vi "Main Program.vi"() -> ()   [LabVIEW 2011]
panel:
  out "Mean Plot":dynamicdata(graph)
  out "Current data plot":cluster{"Y":dbl[], "Y":dbl[]}[](graph)
  in  "UP CONVERSION":enum32{"Set Position ", "Data Accusition"}(tab)
  in  "Position (units)":dbl
  in  "Velocity value (units/s) in":dbl
  out "Current position (units)":dbl
  out "Velocity value (units/s) out":dbl
  in  "stop":bool
  out "Position Time Zero":dbl
  in  "Velocity for detecting position zero":dbl
  in  "Set count 1":i32
  in  "Velocity 1":dbl
  in  "Step Size 1":dbl
  in  "Set count 2":i32
  in  "Velocity 2":dbl
  in  "Step Size 2":dbl
  in  "Set count 3":i32
  in  "Velocity 3":dbl
  in  "Step Size 3":dbl
  in  "Set count 4":i32
  in  "Velocity 4":dbl
  in  "Step Size 4":dbl
  in  "File Path":string="C:\\Users\\nshukla\\Desktop\\2\\"
  in  "Stop Taking Data":bool
  in  "Average file path":path
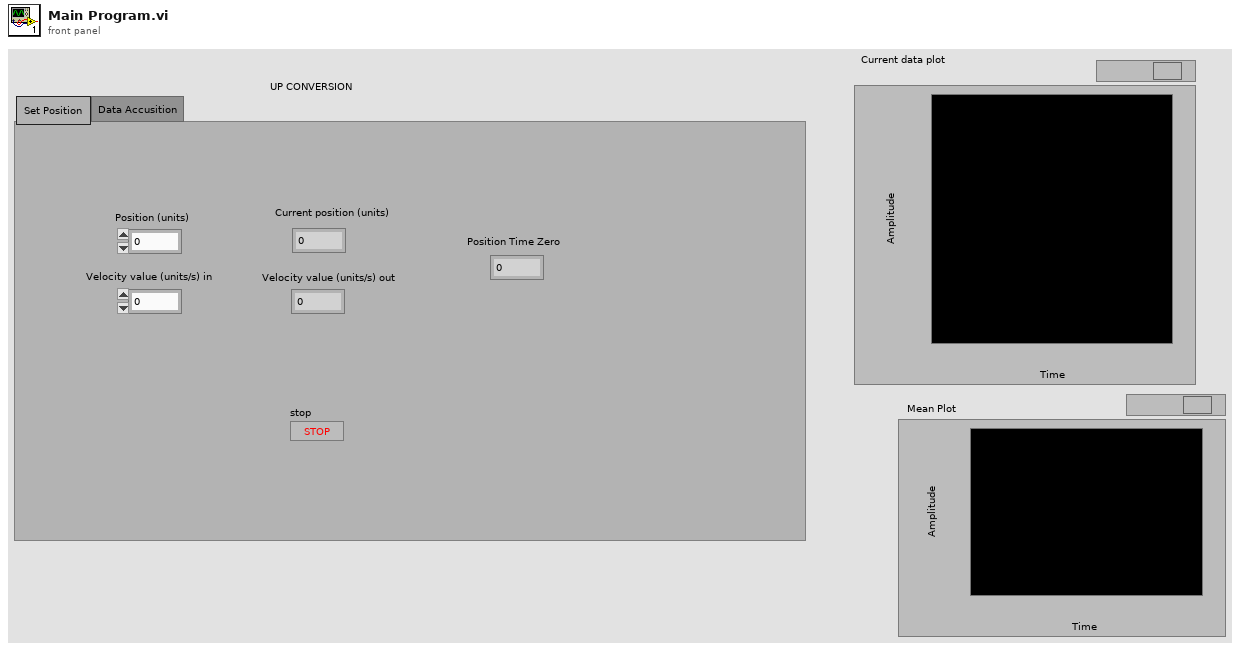
[diagram p1: front panel]
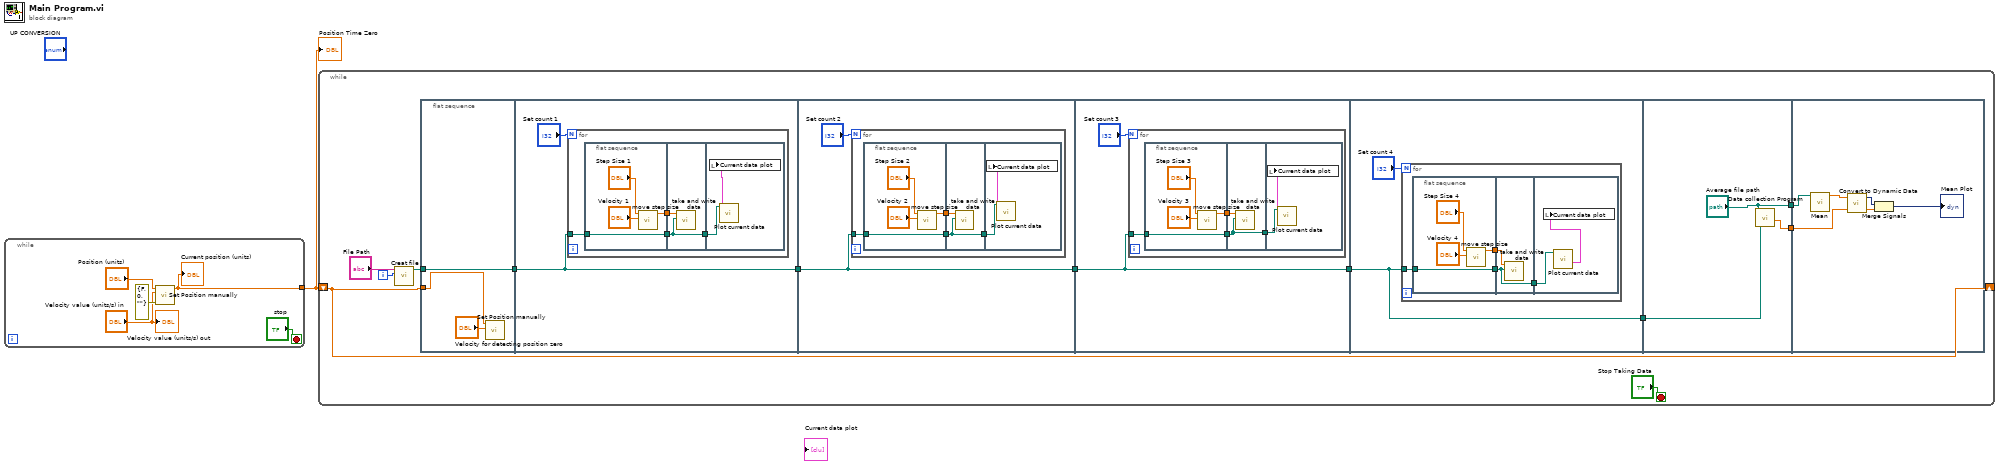
[diagram p0: block diagram]
diagram:
  n1 = while {
    tunnel: [w4] -> w1
    stop <- "stop" stop-if-true
    n2 = call "Set Position manually.vi"("error in (no error)"=errorcluster {"status"=FALSE, "code"=0, "source"=""}, "Velocity value (units/s) in"="Velocity value (units/s) in", "Displacement (units)"="Position (units)") -> ("Current position (units)"=w4:dbl)  [unwired: 7 in, 1 out]
    "Current position (units)" <- w4
    "Velocity value (units/s) out" <- "Velocity value (units/s) in"
  }
  "Position Time Zero" <- w1
  n3 = while {
    shift-right: [w10] -> _
    shift-left: w1 -> [w10]
    i -> [w17]
    stop <- "Stop Taking Data" stop-if-true
    n4 = call "Creat file.vi"("Numeric"=w17, "File Path"="File Path") -> ("Path"=w15:path)  [unwired: 9 in]
    n5 = flat-sequence {
      tunnel: w10 -> [w21]
      tunnel: [w19] -> w16
      tunnel: w15 -> [w19]
      tunnel: w16 -> [w22]
      tunnel: [w22] -> w14
      tunnel: w14 -> [w36]
      tunnel: [w36] -> w12
      tunnel: [w50] -> w13
      tunnel: w12 -> [w50]
      tunnel: w13 -> [w64]
      tunnel: [w64] -> w9
      tunnel: w9 -> [w80]
      tunnel: ["Average file path"] -> w8
      tunnel: [w78] -> w7
      tunnel: w8 -> [w85]
      tunnel: w7 -> [w82]
      frame #0 {
        n6 = call "Set Position manually.vi"("Velocity value (units/s) in"="Velocity for detecting position zero", "Displacement (units)"=w21) -> ()  [unwired: 8 in, 2 out]
      }
      frame #1 {
        n7 = for {
          N: "Set count 1" -> [_]
          tunnel: w22 -> [w25]
          n8 = flat-sequence {
            tunnel: [w29] -> w27
            tunnel: [w28] -> w26
            tunnel: w25 -> [w28]
            tunnel: w27 -> [w33]
            tunnel: w26 -> [w32]
            tunnel: [w32] -> w24
            tunnel: w24 -> [w35]
            frame #0 {
              n9 = call "move step size.vi"("Velocity value (units/s) in"="Velocity 1", "Displacement (units)"="Step Size 1") -> ("Current position (units)"=w29:dbl)  [unwired: 8 in, 1 out]
            }
            frame #1 {
              n10 = call "take and write data.vi"("Path"=w32, "Current position (units)"=w33) -> ()  [unwired: 10 in]
            }
            frame #2 {
              n11 = call "Plot current data.vi"("file path (dialog if empty)"=w35) -> ("XY Graph"=w34:cluster{"Y":dbl[], "Y":dbl[]}[])  [unwired: 10 in]
              n12 = local write "Current data plot"(w34) -> ()
            }
          }
        }
      }
      frame #2 {
        n13 = for {
          N: "Set count 2" -> [_]
          tunnel: w36 -> [w39]
          n14 = flat-sequence {
            tunnel: [w43] -> w41
            tunnel: [w42] -> w40
            tunnel: w39 -> [w42]
            tunnel: w41 -> [w47]
            tunnel: w40 -> [w46]
            tunnel: [w46] -> w38
            tunnel: w38 -> [w49]
            frame #0 {
              n15 = call "move step size.vi"("Velocity value (units/s) in"="Velocity 2", "Displacement (units)"="Step Size 2") -> ("Current position (units)"=w43:dbl)  [unwired: 8 in, 1 out]
            }
            frame #1 {
              n16 = call "take and write data.vi"("Path"=w46, "Current position (units)"=w47) -> ()  [unwired: 10 in]
            }
            frame #2 {
              n17 = call "Plot current data.vi"("file path (dialog if empty)"=w49) -> ("XY Graph"=w48:cluster{"Y":dbl[], "Y":dbl[]}[])  [unwired: 10 in]
              n18 = local write "Current data plot"(w48) -> ()
            }
          }
        }
      }
      frame #3 {
        n19 = for {
          N: "Set count 3" -> [_]
          tunnel: w50 -> [w53]
          n20 = flat-sequence {
            tunnel: [w57] -> w55
            tunnel: [w56] -> w54
            tunnel: w53 -> [w56]
            tunnel: w55 -> [w61]
            tunnel: w54 -> [w60]
            tunnel: [w60] -> w52
            tunnel: w52 -> [w62]
            frame #0 {
              n21 = call "move step size.vi"("Velocity value (units/s) in"="Velocity 3", "Displacement (units)"="Step Size 3") -> ("Current position (units)"=w57:dbl)  [unwired: 8 in, 1 out]
            }
            frame #1 {
              n22 = call "take and write data.vi"("Path"=w60, "Current position (units)"=w61) -> ()  [unwired: 10 in]
            }
            frame #2 {
              n23 = call "Plot current data.vi"("file path (dialog if empty)"=w62) -> ("XY Graph"=w63:cluster{"Y":dbl[], "Y":dbl[]}[])  [unwired: 10 in]
              n24 = local write "Current data plot"(w63) -> ()
            }
          }
        }
      }
      frame #4 {
        n25 = for {
          N: "Set count 4" -> [_]
          tunnel: w64 -> [w67]
          n26 = flat-sequence {
            tunnel: [w71] -> w69
            tunnel: [w70] -> w68
            tunnel: w67 -> [w70]
            tunnel: w69 -> [w75]
            tunnel: w68 -> [w74]
            tunnel: [w74] -> w66
            tunnel: w66 -> [w77]
            frame #0 {
              n27 = call "move step size.vi"("Velocity value (units/s) in"="Velocity 4", "Displacement (units)"="Step Size 4") -> ("Current position (units)"=w71:dbl)  [unwired: 8 in, 1 out]
            }
            frame #1 {
              n28 = call "take and write data.vi"("Path"=w74, "Current position (units)"=w75) -> ()  [unwired: 10 in]
            }
            frame #2 {
              n29 = call "Plot current data.vi"("file path (dialog if empty)"=w77) -> ("XY Graph"=w76:cluster{"Y":dbl[], "Y":dbl[]}[])  [unwired: 10 in]
              n30 = local write "Current data plot"(w76) -> ()
            }
          }
        }
      }
      frame #5 {
        n31 = call "Data collection Program.vi"("Current File Name"=w80, "Average file path"="Average file path") -> ("Numeric"=w78:dbl)  [unwired: 9 in]
      }
      frame #6 {
        n32 = call "Mean.vi"("file path (dialog if empty)"=w85) -> ("Array"=w84:dbl[])  [unwired: 10 in]
        n33 = call "Convert to Dynamic Data"("Array"=w84) -> ("Dynamic Data Type"=w83:dynamicdata)  [unwired: 3 in]
        n34 = Merge Signals(w83, w82) -> (→"Mean Plot":dynamicdata)
      }
    }
  }
